vi "Send Return Synchronize Status.vi"(4 "Status":T1, 6 "error":string, 7 "Message Priority (Normal)":T2=enum."Normal", 8 "error in (no error)":errorcluster, 11 "Message Enqueuer":refnum<class "Message Enqueuer.lvclass">) -> (0 "error out":errorcluster, 3 "Message Enqueuer out":refnum<class "Message Enqueuer.lvclass">)   [LabVIEW 2015, in "SCADA Core.lvlib" / "Return Synchronize Status Msg.lvclass"]
doc: "This VI sends the message to an actor."
uses:
  Return Synchronize Status Msg.lvclass
  <vilib>/ActorFramework/Message Enqueuer/Message Enqueuer.lvclass
  <vilib>/ActorFramework/Message Enqueuer/Message Priority.ctl
  SCADA Abstract Messages/Simple Command Status Msg/Simple Command Status.ctl
  Return Synchronize Status Msg.lvclass/Return Synchronize Status Msg.ctl
  <vilib>/ActorFramework/Message Enqueuer/Message Enqueuer.lvclass/Message Enqueuer.ctl
  <vilib>/ActorFramework/Message Priority Queue/Priority Enqueue.vi
  SCADA Abstract Messages/Simple Command Status Msg/Simple Command Status Msg.lvclass
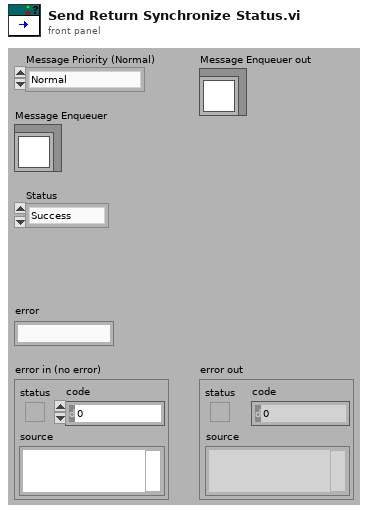
[diagram p1: front panel]
types:
  T1 = typedef "SCADA Core.lvlib/Simple Command Status Msg.lvclass/Simple Command Status.ctl" = enum16{"Success", "Failure"}
  T2 = typedef "Actor Framework.lvlib/Message Enqueuer.lvclass/Message Priority.ctl" = enum16{"Low", "Normal", "High"}
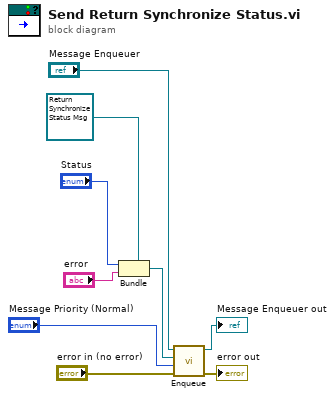
[diagram p0: block diagram]
diagram:
  n1 = Bundle(cluster=refnum<class "Return Synchronize Status Msg.lvclass"> refnum ("Object"), "Status", "error") -> (w5:refnum<class "Return Synchronize Status Msg.lvclass">)
  n2 = call <vilib>:"Enqueue.vi"("error in (no error)"="error in (no error)", "Message Priority (Normal)"="Message Priority (Normal)", "Message"=w5, "Message Enqueuer in"="Message Enqueuer") -> ("error out"=→"error out":errorcluster, "Message Enqueuer out"=→"Message Enqueuer out":refnum<class "Message Enqueuer.lvclass">)  [unwired: 6 in]
